vi "ZLIB Extract__ogtk.vi"   [LabVIEW 2018]
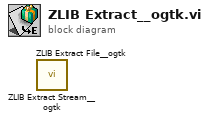
[diagram p0: block diagram]
diagram:
  n1 = call <userlib>:"ZLIB Extract Stream__ogtk.vi"() -> ()  [unwired: 7 in, 3 out]
  n2 = call <userlib>:"ZLIB Extract File__ogtk.vi"() -> ()  [unwired: 8 in, 2 out]
